vi "view -- timer.vi"() -> ()   [LabVIEW 2010]
uses:
  countdown control.ctl
panel:
  out "tic state":enum16{"knock-knock", "none"}(ring)
  in  "Thermometer":dbl(slide) min=2063222878.0 max=2063690576.0 scale=0.0..100.0
  in  "interval (sec)":dbl=10.0
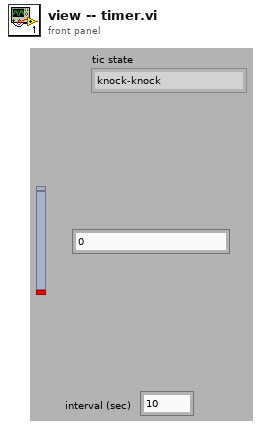
[diagram p1: front panel]
types:
  T1 = typedef "countdown control.ctl" = enum16{"check", "start", "reset"}
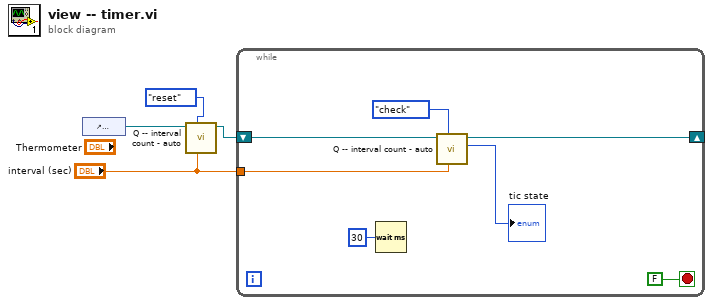
[diagram p0: block diagram]
diagram:
  n1 = control-ref of="Thermometer"() -> (w2:refnum<vi>)
  n2 = call "Q -- interval count - auto.vi"("interval (sec)"="interval (sec)", "action"=countdown_control."reset", "timer ref"=w2) -> ("timer out"=w3:refnum<vi>)  [unwired: 6 in, 2 out]
  n3 = while {
    shift-right: [w8] -> _
    shift-left: w3 -> [w9]
    tunnel: "interval (sec)" -> [w5]
    stop <- FALSE stop-if-true
    n4 = Wait (ms)(milliseconds to wait=u32 30) -> ()  [unwired: 1 out]
    n5 = call "Q -- interval count - auto.vi"("interval (sec)"=w5, "action"=countdown_control."check", "timer ref"=w9) -> ("tic state"=→"tic state":enum16{"knock-knock", "none"}, "timer out"=w8:refnum<vi>)  [unwired: 6 in, 1 out]
  }
